vi "timeout--fgv.vi"(6 "Module ID":i32=-1, 7 "Action":T1, 11 "Module Timeout in":i32) -> (3 "Module Timeout out":i32)   [LabVIEW 2022 SP3, in "hse-db.lvlib" / "DB_CONNECTOR.lvlib"]
doc: "Extends the functionality of 'Module Timeout--constant.vi'.\nThe Module Timeout value can be overriden with a request.\nThe current value is stored inside this FGV per clonable.\nThe Module Timeout value must be greater 0, otherwise a default value of 5000 is used.\n\n____\nHAMPEL SOFTWARE ENGINEERING v1.4.0 (2023-12-19 09:52)"
uses:
  DB_CONNECTOR.lvlib
  timeout-fgv-actions--control.ctl
panel:
  # "Connector Pane"
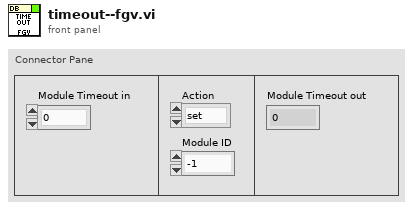
[diagram p1: front panel]
types:
  T1 = typedef "hse-db.lvlib/DB_CONNECTOR.lvlib/timeout-fgv-actions--control.ctl" = enum16{"set", "get"}
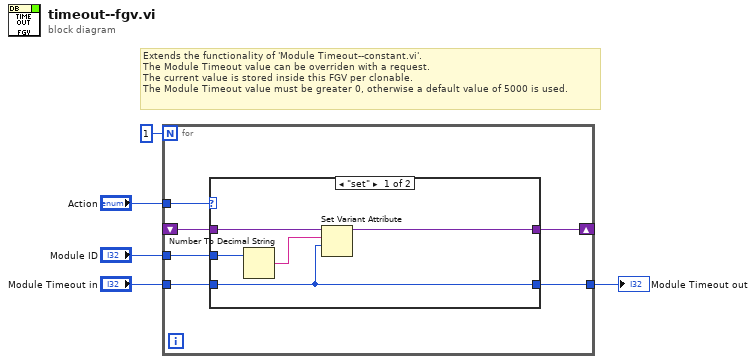
[diagram p0: block diagram]
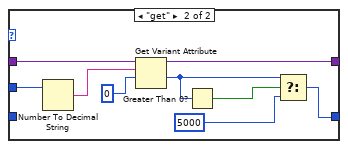
[diagram p2: hidden frame]
diagram:
  # "Extends the functionality of 'Module Timeout--constant.vi'.\nThe Module Timeout value can be overriden with a request.\nThe current value is stored inside this FGV per clonable.\nThe Module Timeout value must be greater 0, otherwise a default value of 5000 is used."
  n1 = for {
    N: 1 -> [_]
    tunnel: "Action" -> [w11]
    shift-right: [w10] -> _
    shift-left: _ -> [w9]
    tunnel: "Module ID" -> [w8]
    tunnel: "Module Timeout in" -> [w7]
    tunnel: [w6] -> w2
    n2 = case shown="\"set\"" w11 {
      tunnel: [w15 w24] -> w10
      tunnel: w9 -> [w16 w25]
      tunnel: w8 -> [w14 w23]
      tunnel: w7 -> [w12 _]
      tunnel: [w12 w17] -> w6
      frame "set" {
        n3 = Number To Decimal String(number=w14) -> (decimal integer string=w13:string)  [unwired: 1 in]
        n4 = Set Variant Attribute(Variant=w16, name=w13, value=w12) -> (Variant out=w15:variant)  [unwired: 1 in, 2 out]
      }
      frame "get" {
        n5 = Number To Decimal String(number=w23) -> (decimal integer string=w22:string)  [unwired: 1 in]
        n6 = Get Variant Attribute(Variant=w25, name=w22, default value (empty Variant)=0 ("Module Timeout out")) -> (duplicate Variant=w24:variant, value=w19:i32)  [unwired: 1 in, 2 out]
        n7 = Greater Than 0?(x=w19) -> (x > 0?=w20:bool)
        n8 = Select(t=w19, s=w20, f=5000) -> (s? t:f=w17:i32)
      }
    }
  }
  "Module Timeout out" <- w2
